vi "Parse Cluster Variant.vi"(9 "Cluster Variant in":variant, 10 "Group Parameters in":string) -> (1 "appended array":variant[](array[variant]), 2 "Group Parameters out":string[](array[string]))   [LabVIEW 2019, in "TDMS.lvlib" / "TDMS.lvclass"]
uses:
  TDMS.lvclass
  <vilib>/Utility/VariantDataType/VariantType.lvlib
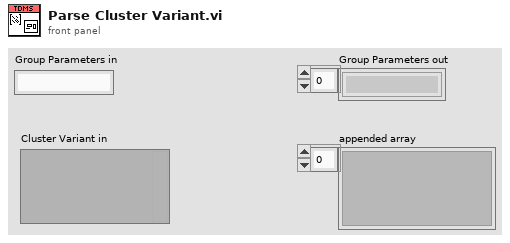
[diagram p1: front panel]
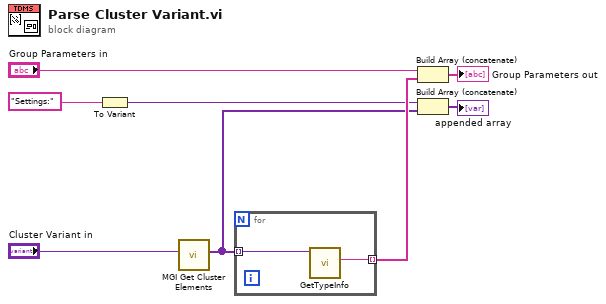
[diagram p0: block diagram]
diagram:
  n1 = To Variant(anything="Settings:") -> (Variant=w4:variant)
  n2 = call <userlib>:"MGI Get Cluster Elements.vi"("Cluster"="Cluster Variant in") -> ("Cluster Elements"=w3:variant[])  [unwired: 9 in, 1 out]
  n3 = for {
    tunnel: w3 -> [w10] mode=indexing
    tunnel: [w9] -> w6 mode=indexing
    n4 = call <vilib>:"GetTypeInfo.vi"("Variant"=w10) -> ("Name"=w9:string)  [unwired: 6 in, 4 out]
  }
  n5 = Build Array (concatenate)("Group Parameters in", w6) -> (→"Group Parameters out":string[])
  n6 = Build Array (concatenate)(w4, w3) -> (→"appended array":variant[])
